vi "12x12 Mapping Data Plot.vi"() -> ()   [LabVIEW 2012]
uses:
  <vilib>/Utility/miscctls.llb/LVPointDoubleTypeDef.ctl
panel:
  out "Counts under curve":dbl[][](array[numeric])=[[0.0, 105.0, 108.0, 96.0, 96.0, 91.0, 85.0], [0.0, 133.0, 105.0, 97.0, 115.0, 96.0, 86.0], [0.0, 257.0, 244.0, 227.0, 195.0, 194.0, 94.0], [0.0, 255.0, 253.0, 258.0, 293.0, 296.0, 96.0], [0.0, 125.0, 160.0, 164.0, 196.0, 206.0, 83.0], [0.0, 107.0, 106.0, 102.0, 94.0, 103.0, 99.0]]
  in  "Cursor.Cursor Position 2":T1
  in  "peak centerRcm-1":dbl=519.0
  in  "peak widthRcm-1":dbl=8.0
  out "error out":errorcluster
  out "Raman Map":dbl[][](graph)
  in  "stop":bool
  out "plot graph":cluster{"Y":dbl[], "Y":dbl[]}[](graph)
  in  "Path":path=path "E:/Documents/lab/Maps"
  in  "2 Letter File Name":string="QS"
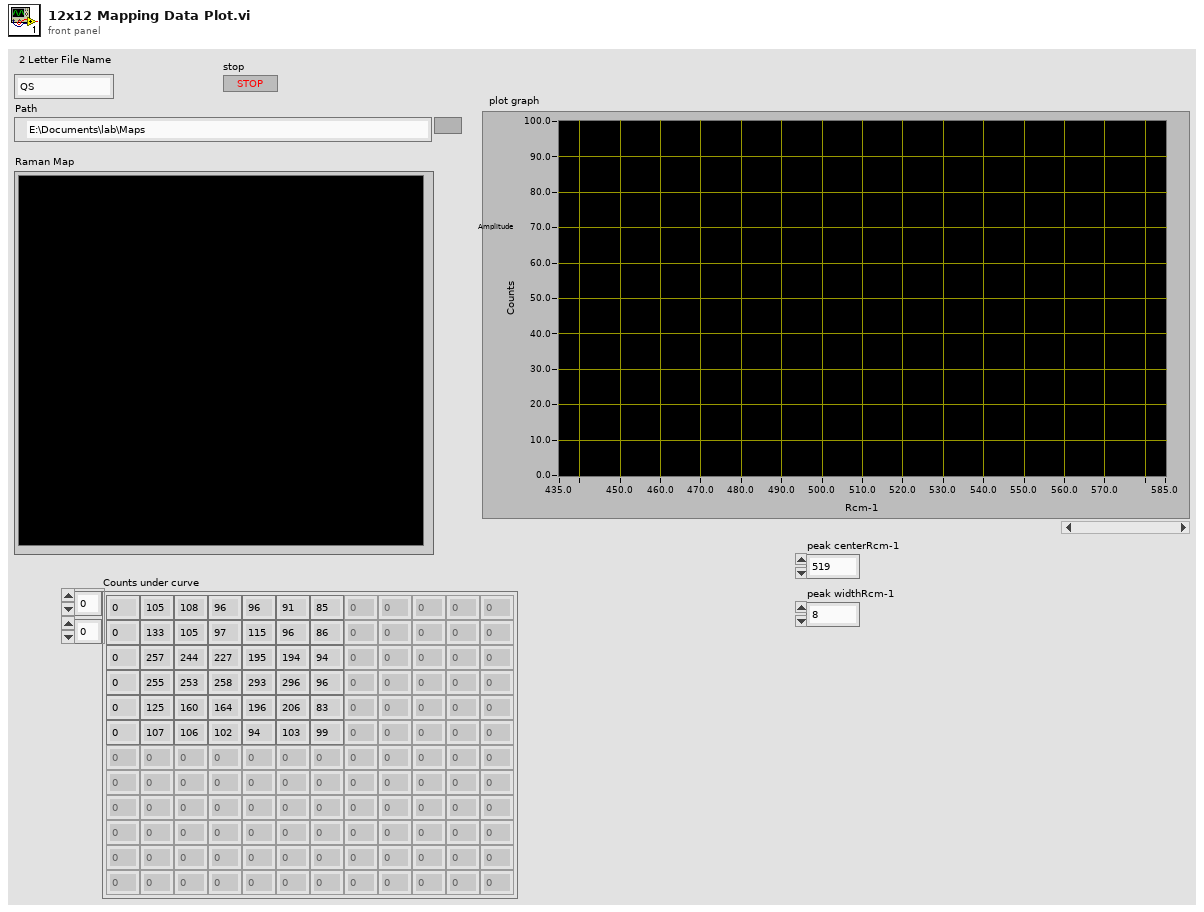
[diagram p1: front panel]
types:
  T1 = typedef "LVPointDoubleTypeDef.ctl" = cluster{"X":dbl, "Y":dbl}
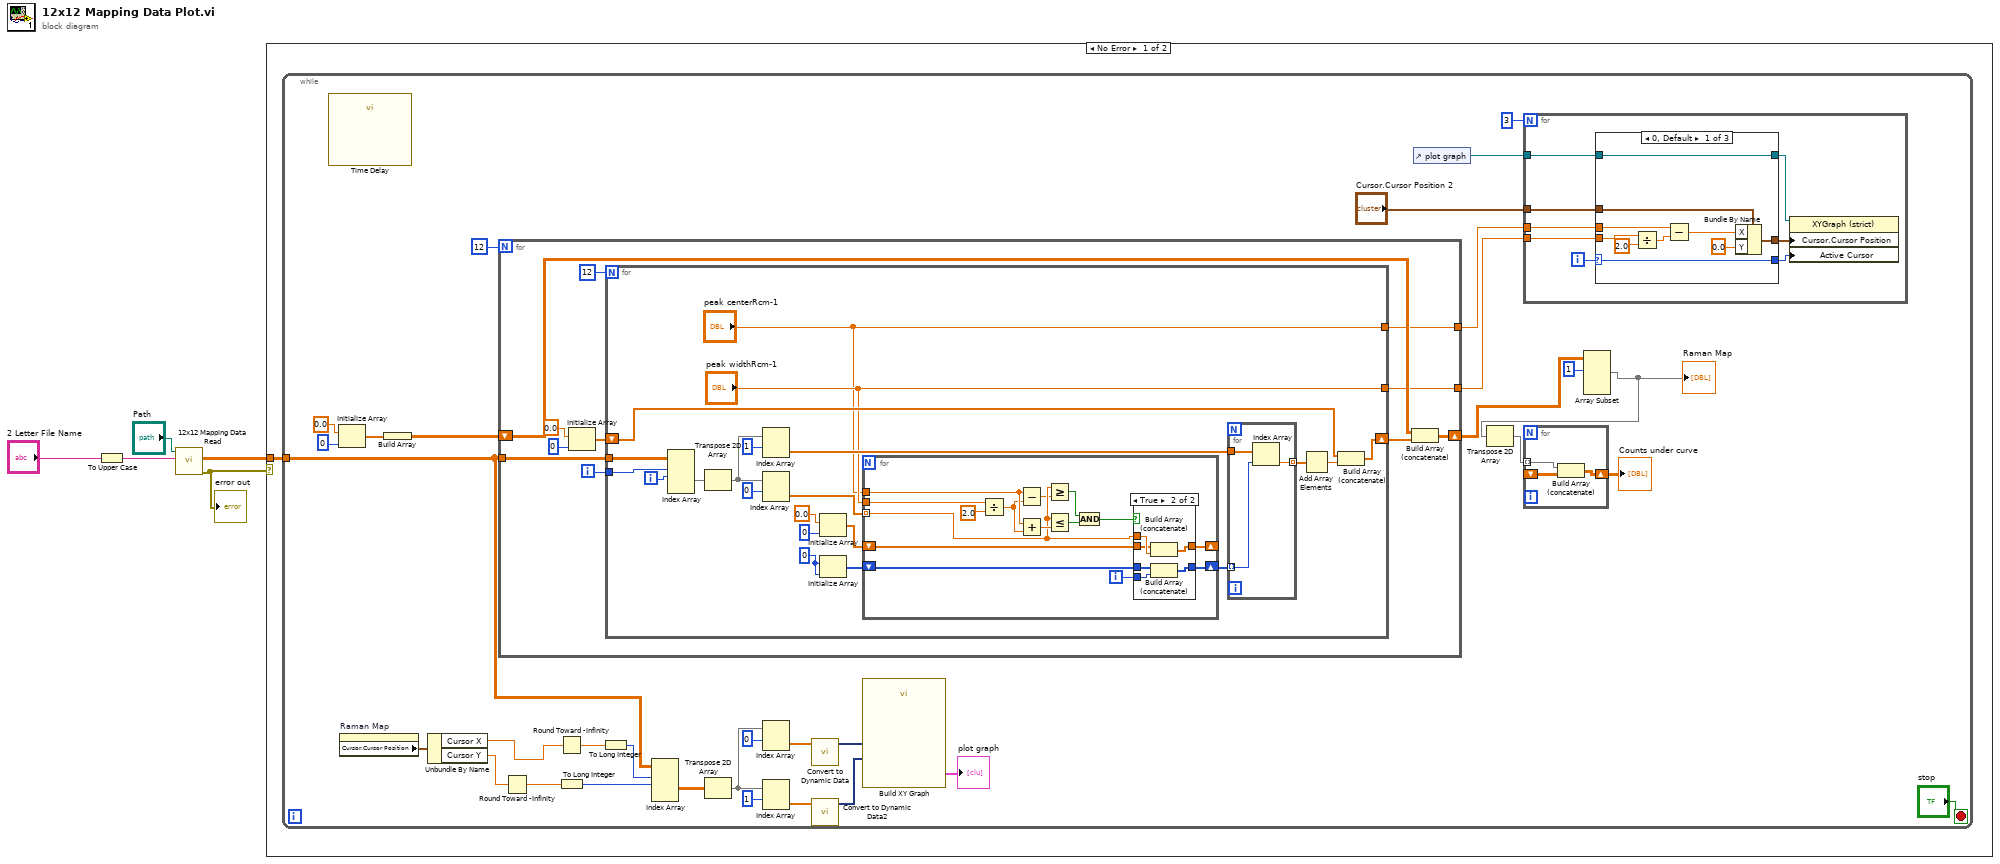
[diagram p0: block diagram]
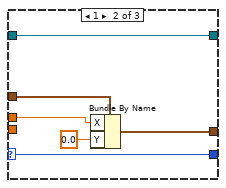
[diagram p2: hidden frame]
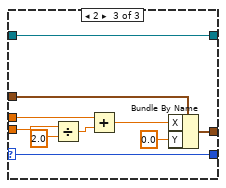
[diagram p3: hidden frame]
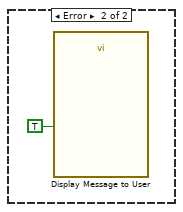
[diagram p5: hidden frame]
diagram:
  n1 = To Upper Case(1:"2 Letter File Name") -> (0:w1:string)
  n2 = call "12x12 Mapping Data Read.vi"("Small File name"=w1, "Path"="Path") -> ("error out"=w3:errorcluster, "all rows"=w4:dbl[][][][])  [unwired: 8 in]
  "error out" <- w3
  n3 = case shown="No Error" w3 {
    tunnel: w4 -> [w6 _]
    frame No Error {
      n4 = while {
        tunnel: w6 -> [w30]
        stop <- "stop" stop-if-true
        n5 = call "Time Delay"() -> ()  [unwired: 11 in, 1 out]
        n6 = Initialize Array(0.0 ("element"), 0 ("dimension size")) -> (w26:dbl[])
        n7 = property on="Raman Map" class="IntGraph (strict)"() -> ("Cursor.Cursor Position"=w13:T1)  [unwired: 2 in, 2 out]
        n8 = Build Array(w26) -> (w25:dbl[][])
        n9 = Unbundle By Name(w13) -> ("Cursor X"=w8:dbl, "Cursor Y"=w16:dbl)
        n10 = for {
          N: 12 -> [_]
          tunnel: w30 -> [w87]
          shift-right: [w79] -> w9
          shift-left: w25 -> [w80]
          tunnel: [w78] -> w23
          tunnel: [w77] -> w19
          i -> [w86]
          n11 = Initialize Array(0.0 ("element"), 0 ("dimension size")) -> (w82:dbl[])
          n12 = for {
            N: 12 -> [_]
            tunnel: w87 -> [w99]
            tunnel: w86 -> [w98]
            shift-right: [w91] -> w81
            shift-left: w82 -> [w90]
            tunnel: ["peak centerRcm-1"] -> w78
            tunnel: ["peak widthRcm-1"] -> w77
            i -> [w93]
            w102 = 0 ("dimension size")
            n13 = Index Array(array=w99, index (dim 0)=w98, index (dim 1)=w93) -> (element=w100:dbl[][])  [unwired: 2 in]
            n14 = Transpose 2D Array(2D array=w100) -> (transposed array=w96:dbl[][])
            n15 = Index Array(array=w96, index (row)=1) -> (element=w94:dbl[])  [unwired: 1 in]
            n16 = Index Array(array=w96, index (row)=0) -> (element=w107:dbl[])  [unwired: 1 in]
            n17 = Initialize Array(0.0 ("element"), 0 ("dimension size")) -> (w105:dbl[])
            n18 = Initialize Array(w102, w102) -> (w103:i32[])
            n19 = for {
              tunnel: w107 -> [w122] mode=indexing
              shift-right: [w119] -> _
              shift-left: w105 -> [w120]
              shift-right: [w118] -> w97
              shift-left: w103 -> [w117]
              tunnel: "peak centerRcm-1" -> [w116]
              tunnel: "peak widthRcm-1" -> [w114]
              i -> [w121]
              n20 = Divide(x=w114, y=2.0) -> (x/y=w112:dbl)
              n21 = Subtract(x=w116, y=w112) -> (x-y=w113:dbl)
              n22 = Add(x=w116, y=w112) -> (x+y=w126:dbl)
              n23 = Greater Or Equal?(x=w122, y=w113) -> (x >= y?=w125:bool)
              n24 = Less Or Equal?(x=w122, y=w126) -> (x <= y?=w124:bool)
              n25 = And(x=w125, y=w124) -> (x .and. y?=w123:bool)
              n26 = case shown="True" w123 {
                tunnel: w122 -> [_ w134]
                tunnel: w121 -> [_ w131]
                tunnel: w120 -> [w128 w133]
                tunnel: [w128 w132] -> w119
                tunnel: [w127 w130] -> w118
                tunnel: w117 -> [w127 w129]
                frame False {
                }
                frame True {
                  n27 = Build Array (concatenate)(w133, w134) -> (w132:dbl[])
                  n28 = Build Array (concatenate)(w129, w131) -> (w130:i32[])
                }
              }
            }
            n29 = for {
              tunnel: w97 -> [w111] mode=indexing
              tunnel: [w110] -> w101 mode=indexing
              tunnel: w94 -> [w109]
              n30 = Index Array(array=w109, index=w111) -> (element=w110:dbl)
            }
            n31 = Add Array Elements(numeric array=w101) -> (sum=w92:dbl)
            n32 = Build Array (concatenate)(w90, w92) -> (w91:dbl[])
          }
          n33 = Build Array (concatenate)(w80, w81) -> (w79:dbl[][])
        }
        n34 = Round Toward -Infinity(1:w16) -> (0:w12:dbl)
        n35 = Round Toward -Infinity(1:w8) -> (0:w11:dbl)
        n36 = To Long Integer(number=w12) -> (32bit integer=w15:i32)
        n37 = To Long Integer(number=w11) -> (32bit integer=w14:i32)
        n38 = Index Array(array=w30, index (dim 0)=w14, index (dim 1)=w15) -> (element=w39:dbl[][])  [unwired: 2 in]
        n39 = Transpose 2D Array(2D array=w39) -> (transposed array=w38:dbl[][])
        n40 = Index Array(array=w38, index (row)=0) -> (element=w31:dbl[])  [unwired: 1 in]
        n41 = Index Array(array=w38, index (row)=1) -> (element=w28:dbl[])  [unwired: 1 in]
        n42 = call "Convert to Dynamic Data"("Array"=w31) -> ("Dynamic Data Type"=w34:dynamicdata)  [unwired: 3 in]
        n43 = call "Convert to Dynamic Data2"("Array"=w28) -> ("Dynamic Data Type"=w33:dynamicdata)  [unwired: 3 in]
        n44 = call "Build XY Graph"("Y Input"=w33, "X Input"=w34) -> ("XY Graph"=→"plot graph":cluster{"Y":dbl[], "Y":dbl[]}[])  [unwired: 3 in, 6 out]
        n45 = control-ref of="plot graph"() -> (w20:refnum<vi>)
        n46 = for {
          N: 3 -> [_]
          tunnel: w23 -> [w43]
          tunnel: "Cursor.Cursor Position 2" -> [w49]
          tunnel: w20 -> [w48]
          tunnel: w19 -> [w47]
          i -> [w50]
          n47 = case shown="0, Default" w50 {
            selector: w50 -> [w59 w61 w75]
            tunnel: w43 -> [w53 w65 w70]
            tunnel: w49 -> [w57 w64 w73]
            tunnel: w48 -> [w60 w63 w76]
            tunnel: w47 -> [w54 _ w71]
            tunnel: [w60 w63 w76] -> w46
            tunnel: [w58 w62 w74] -> w45
            tunnel: [w59 w61 w75] -> w44
            frame 0, Default {
              n48 = Divide(x=w54, y=2.0) -> (x/y=w52:dbl)
              n49 = Subtract(x=w53, y=w52) -> (x-y=w51:dbl)
              n50 = Bundle By Name(cluster=w57, "X"=w51, "Y"=0.0) -> (w58:T1)
            }
            frame 1 {
              n51 = Bundle By Name(cluster=w64, "X"=w65, "Y"=0.0) -> (w62:T1)
            }
            frame 2 {
              n52 = Divide(x=w71, y=2.0) -> (x/y=w69:dbl)
              n53 = Add(x=w70, y=w69) -> (x+y=w68:dbl)
              n54 = Bundle By Name(cluster=w73, "X"=w68, "Y"=0.0) -> (w74:T1)
            }
          }
          n55 = property class="XYGraph (strict)"(reference=w46, "Cursor.Cursor Position"=w45, "Active Cursor"=w44) -> ()  [unwired: 1 in, 2 out]
        }
        n56 = Array Subset(array=w9, index (row)=1 ("index")) -> (w7:dbl[][])  [unwired: 3 in]
        "Raman Map" <- w7
        n57 = Transpose 2D Array(2D array=w7) -> (transposed array=w18:dbl[][])
        n58 = for {
          tunnel: w18 -> [w40] mode=indexing
          shift-right: [w42] -> w17
          shift-left: _ -> [w41]
          n59 = Build Array (concatenate)(w40, w41) -> (w42:dbl[][])
        }
        "Counts under curve" <- w17
      }
    }
    frame Error {
      n60 = call "Display Message to User"("Enable"=TRUE) -> ()  [unwired: 9 in, 2 out]
    }
  }
